vi "DriveModuleControlLogic_ORIG.vi"(8 "Pass_Through_Time":dbl=-1.0 format="%33.4f", 9 "Actual State":T1 {"Angle"."SIN" format="%13.4f"; "Angle"."COS" format="%13.4f"; "Angle"."VALUE" format="%13.4f"}, 10 "Desired State":T1={"Speed"=0.0, "Angle"={"VALUE"=0.0, "COS"=1.0, "SIN"=0.0}} {"Angle"."SIN" format="%13.4f"; "Angle"."COS" format="%13.4f"; "Angle"."VALUE" format="%13.4f"}, 11 "ModualNamePrefix":i32) -> (2 "SpinMotorDmd":dbl, 3 "TravelMotorDmd":dbl)   [LabVIEW 2023]
uses:
  <vilib>/Rock Robotics/WPI/ThirdParty/JAS_Junk/TrajLib/TypeDef/SWERVE_DRIVE_MODULE_STATE.ctl
  <vilib>/Rock Robotics/WPI/ThirdParty/JAS_Junk/TrajLib/TypeDef/ROTATION2D.ctl
  <vilib>/Rock Robotics/WPI/ThirdParty/JAS_Junk/TrajLib/Rotation2d_Minus.vi
  <vilib>/Rock Robotics/WPI/ThirdParty/JAS_Junk/TrajLib/Rotation2d_GetRadians.vi
  <vilib>/Rock Robotics/WPI/ThirdParty/JAS_Junk/TrajLib/SwerveModuleState_New.vi
  <vilib>/Rock Robotics/WPI/ThirdParty/JAS_Junk/TrajLib/Rotation2d_RotateBy.vi
  <vilib>/Rock Robotics/WPI/ThirdParty/JAS_Junk/TrajLib/Rotation2d_CreateAngle.vi
  <vilib>/Rock Robotics/WPI/ThirdParty/JAS_Junk/TrajLib/SimpleMotorFF_Calculate.vi
  <vilib>/Rock Robotics/WPI/ThirdParty/JAS_Junk/TrajLib/PIDController_AtSetpoint.vi
  <vilib>/Rock Robotics/WPI/ThirdParty/JAS_Junk/TrajLib/PIDController_SetPIDF.vi
  <vilib>/Rock Robotics/WPI/ThirdParty/JAS_Junk/TrajLib/PIDController_SetDerivativeFilter.vi
  <vilib>/Rock Robotics/WPI/ThirdParty/JAS_Junk/TrajLib/PIDController_SetIntegratorRange.vi
  <vilib>/Rock Robotics/WPI/ThirdParty/JAS_Junk/TrajLib/PIDController_SetTolerancePandV.vi
  <vilib>/Rock Robotics/WPI/ThirdParty/JAS_Junk/TrajLib/PIDController_DisableContinousInput.vi
  <vilib>/Rock Robotics/WPI/ThirdParty/JAS_Junk/TrajLib/PIDController_EnableContinousInput.vi
  <vilib>/Rock Robotics/WPI/ThirdParty/JAS_Junk/TrajLib/PIDController_Reset.vi
  <vilib>/Rock Robotics/WPI/ThirdParty/JAS_Junk/TrajLib/PIDController_New.vi
  <vilib>/Rock Robotics/WPI/ThirdParty/JAS_Junk/TrajLib/PIDController_SetOutputLimits.vi
  <vilib>/Rock Robotics/WPI/ThirdParty/JAS_Junk/TrajLib/VI/PIDController_SetIntegratorZone.vi
  <vilib>/Rock Robotics/WPI/ThirdParty/JAS_Junk/TrajLib/SlewRateLimiter_New.vi
  <vilib>/Rock Robotics/WPI/ThirdParty/JAS_Junk/TrajLib/SlewRateLimiter_Reset.vi
  <vilib>/Rock Robotics/WPI/ThirdParty/JAS_Junk/TrajLib/SlewRateLimiter_Calculate.vi
  <vilib>/Rock Robotics/WPI/ThirdParty/JAS_Junk/TrajLib/SlewRateLimiter_SetRate.vi
  <vilib>/Rock Robotics/WPI/ThirdParty/JAS_Junk/TrajLib/VI/Util_GetTime_U32.vi
  <vilib>/Rock Robotics/WPI/ThirdParty/JAS_Junk/TrajLib/MathUtil_Clamp.vi
  <vilib>/Rock Robotics/WPI/ThirdParty/JAS_Junk/TrajLib/VI/MathUtil_RateOfChange.vi
  <vilib>/Rock Robotics/WPI/ThirdParty/JAS_Junk/TrajLib/Rotation2d_UnaryMinus.vi
  <vilib>/Rock Robotics/WPI/ThirdParty/JAS_Junk/TrajLib/Rotation2d_CreateXY.vi
  <vilib>/Rock Robotics/WPI/ThirdParty/JAS_Junk/TrajLib/PIDController_NewPeriod.vi
  <vilib>/Rock Robotics/WPI/ThirdParty/JAS_Junk/TrajLib/Util_CalcDist.vi
  <vilib>/Rock Robotics/SystemInterfaces/NetworkCommunication/NetComm_UsageReport_report.vi
  Robot Global Data.vi
  DriveGlobal.vi
  <vilib>/Rock Robotics/WPI/ThirdParty/JAS_Junk/TrajLib/VI/Util_GetTime_U64.vi
  <vilib>/Rock Robotics/WPI/ThirdParty/JAS_Junk/TrajLib/Globals/Util_LibraryGlobals.vi
  <vilib>/Rock Robotics/WPI/ThirdParty/JAS_Junk/TrajLib/PIDController_AdvCalculate_FF_Sp_Pv.vi
  <vilib>/Rock Robotics/WPI/ThirdParty/JAS_Junk/TrajLib/Trajectory_Library.lvlib
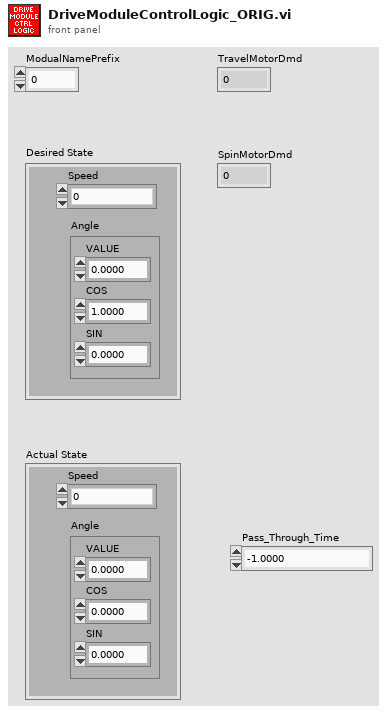
[diagram p1: front panel]
types:
  T1 = typedef "Trajectory_Library.lvlib/SWERVE_DRIVE_MODULE_STATE.ctl" = cluster{"Speed":dbl, "Angle":T2}
  T2 = typedef "Trajectory_Library.lvlib/ROTATION2D.ctl" = cluster{"VALUE":dbl, "COS":dbl, "SIN":dbl}
  T3 = typedef "Trajectory_Library.lvlib/SIMPLE_MOTOR_FF.ctl" = cluster{"Ks":dbl, "Kv":dbl, "Ka":dbl, "KnInv":dbl}
  T4 = typedef "Trajectory_Library.lvlib/PID_ADV_LIMITS.ctl" = cluster{"MaxInput":dbl, "MinInput":dbl, "Continuous":bool, "MaxOutput":dbl, "MinOutput":dbl}
  T5 = typedef "Trajectory_Library.lvlib/PID_ADV_TUNING.ctl" = cluster{"Kf":dbl, "Kp":dbl, "Ki":dbl, "Kd":dbl, "MaximumIntegral":dbl, "MinimumIntegral":dbl, "Filter Derivative":bool, "IntegralZone":dbl}
  T6 = typedef "Trajectory_Library.lvlib/PosCtrl_Tuning_Type.ctl" = cluster{"Slope":dbl, "Offset":dbl, "Error Deadband":dbl, "At Reference Count":i32, "Negate Output":bool, "Max Allowd Position":dbl, "Min Allowd Position":dbl, "Kd":dbl, "FilterDerivative":bool}
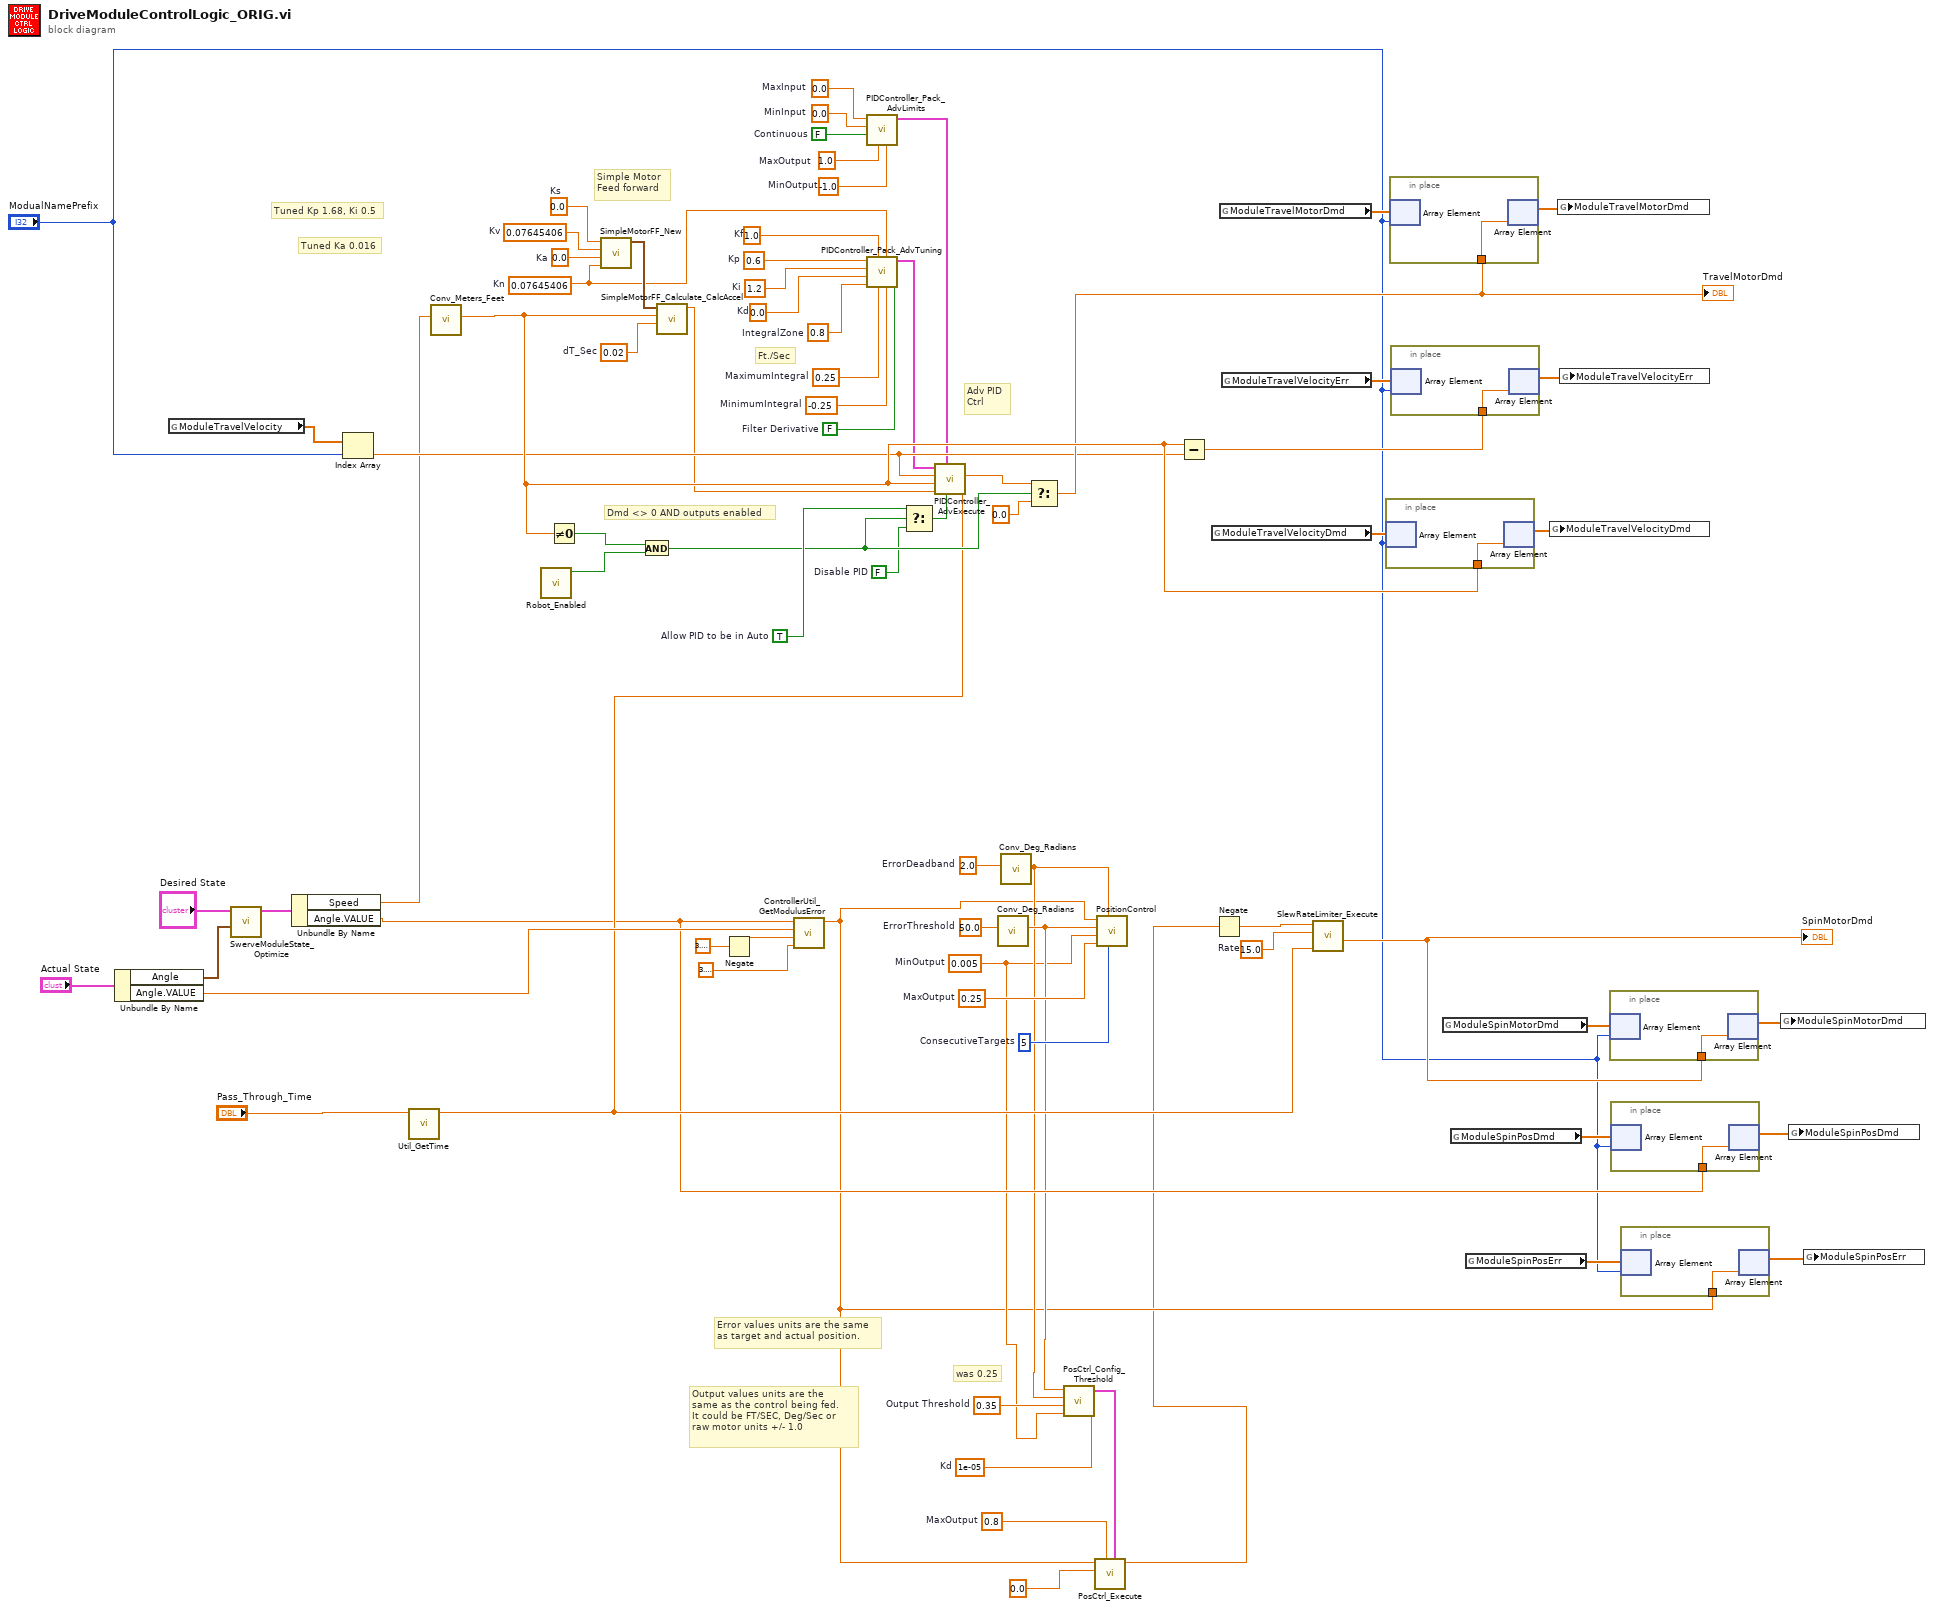
[diagram p0: block diagram]
diagram:
  w10 = 1e-05  # Kd
  w9 = 0.8  # MaxOutput
  w7 = 0.35  # Output Threshold
  w12 = 0.8  # IntegralZone
  w64 = 15.0  # Rate
  w63 = TRUE  # Allow PID to be in Auto
  w61 = FALSE  # Disable PID
  w40 = 0.6  # Kp
  w41 = 1.2  # Ki
  w42 = 0.0  # Kd
  w43 = 1.0  # Kf
  w44 = 0.25  # MaximumIntegral
  w45 = -0.25  # MinimumIntegral
  w46 = FALSE  # Filter Derivative
  w48 = 0.0  # MinInput
  w49 = FALSE  # Continuous
  w50 = 1.0  # MaxOutput
  w47 = -1.0  # MinOutput
  w51 = 0.0  # MaxInput
  w11 = 0.07645406  # Kn
  w35 = 0.02  # dT_Sec
  w37 = 0.0  # Ks
  w38 = 0.07645406  # Kv
  w39 = 0.0  # Ka
  w30 = 5  # ConsecutiveTargets
  w31 = 0.25  # MaxOutput
  w4 = 0.005  # MinOutput
  w33 = 50.0  # ErrorThreshold
  w32 = 2.0  # ErrorDeadband
  # "was 0.25"
  # "Output values units are the\nsame as the control being fed.  \nIt could be FT/SEC, Deg/Sec or\nraw motor units +/- 1.0"
  # "Error values units are the same \nas target and actual position."
  # "Ft./Sec"
  # "Tuned Kp 1.68, Ki 0.5"
  # "Tuned Ka 0.016"
  # "Dmd <> 0 AND outputs enabled"
  # "Adv PID\nCtrl"
  # "Simple Motor\nFeed forward"
  n1 = Unbundle By Name("Actual State") -> ("Angle"=w24:T2, "Angle.VALUE"=w27:dbl)
  n2 = global read "DriveGlobal.vi" "ModuleTravelVelocity"() -> (w55:dbl[])
  n3 = call <vilib>:"SwerveModuleState_Optimize.vi"("CurrentAngle"=w24, "Desired State"="Desired State") -> ("out SWERVE_DRIVE_MODULE_STATE"=w26:T1)  [unwired: 9 in]
  n4 = Unbundle By Name(w26) -> ("Speed"=w34:dbl, "Angle.VALUE"=w16:dbl)
  n5 = Index Array(array=w55, index="ModualNamePrefix") -> (element=w56:dbl)
  n6 = call <vilib>:"Util_GetTime.vi"("Pass_Through_Time"="Pass_Through_Time") -> ("FPGA_Time_Seconds"=w21:dbl)  [unwired: 8 in, 2 out]
  n7 = call <vilib>:"Conv_Meters_Feet.vi"("Meters"=w34) -> ("Feet"=w74:dbl)  [unwired: 10 in]
  n8 = call "Robot_Enabled.vi"() -> ("Robot Enabled"=w19:bool)  [unwired: 11 in]
  n9 = Not Equal To 0?(x=w74) -> (x != 0?=w59:bool)
  n10 = call <vilib>:"SimpleMotorFF_New.vi"("Kn"=w11, "Ka"=w39, "Kv"=w38, "Ks"=w37) -> ("SIMPLE_MOTOR_FF"=w36:T3)  [unwired: 7 in]
  n11 = And(x=w59, y=w19) -> (x .and. y?=w62:bool)
  n12 = call <vilib>:"SimpleMotorFF_Calculate_CalcAccel.vi"("dT_Sec"=w35, "VelSp"=w74, "SIMPLE_MOTOR_FF"=w36) -> ("FeedForward"=w54:dbl)  [unwired: 8 in]
  n13 = Negate(x=3.141592653589793) -> (-x=w25:dbl)
  n14 = call <vilib>:"ControllerUtil_GetModulusError.vi"("Maximum_Input"=3.141592653589793, "Minimum_Input"=w25, "Measurerment(PV)"=w27, "Reference(SP)"=w16) -> ("Error"=w3:dbl)  [unwired: 7 in]
  n15 = call <vilib>:"PIDController_Pack_AdvLimits.vi"("MinOutput"=w47, "MaxOutput"=w50, "Continuous"=w49, "MinInput"=w48, "MaxInput"=w51) -> ("Adv PID Limits"=w53:T4)  [unwired: 6 in]
  n16 = call <vilib>:"PIDController_Pack_AdvTuning.vi"("Filter Derivative"=w46, "MinimumIntegral"=w45, "Kn"=w11, "MaximumIntegral"=w44, "Kf"=w43, "IntegralZone"=w12, "Kd"=w42, "Ki"=w41, "Kp"=w40) -> ("Adv PID Tuning"=w52:T5)  [unwired: 2 in]
  n17 = Select(t=w63, s=w62, f=w61) -> (s? t:f=w60:bool)
  n18 = call <vilib>:"PIDController_AdvExecute.vi"("Time"=w21, "Auto"=w60, "Adv PID Limits"=w53, "FF-FeedForward"=w54, "SP-SetPoint"=w74, "PV-Measurement"=w56, "Adv PID Tuning"=w52) -> ("CO-ControlOutput"=w57:dbl)  [unwired: 2 in, 2 out]
  n19 = call <vilib>:"Conv_Deg_Radians.vi"("Degress"=w33) -> ("Radians"=w6:dbl)  [unwired: 10 in]
  n20 = call <vilib>:"Conv_Deg_Radians.vi"("Degress"=w32) -> ("Radians"=w5:dbl)  [unwired: 10 in]
  n21 = Select(t=w57, s=w62, f=0.0 ("t")) -> (s? t:f=w68:dbl)
  "TravelMotorDmd" <- w68
  n22 = call <vilib>:"PosCtrl_Config_Threshold.vi"("Kd"=w10, "Output Deadband"=w4, "Output Threshold"=w7, "ErrorDeadband"=w5, "ErrorThreshold"=w6) -> ("PosCtrl_Config_Params"=w8:T6)  [unwired: 5 in, 1 out]
  n23 = call <vilib>:"PosCtrl_Execute.vi"("PosCtrl_Config_Params"=w8, "MaxOutput"=w9, "CurrentPosition"=0.0, "TargetPosition"=w3) -> ("Output"=w1:dbl)  [unwired: 5 in, 2 out]
  n24 = call "PositionControl.vi"("ConsecutiveTargets"=w30, "ErrorDeadband"=w5, "MaxOutput"=w31, "MinOutput"=w4, "ErrorThreshold"=w6, "Error"=w3) -> ()  [unwired: 3 in, 3 out]
  n25 = Subtract(x=w74, y=w56) -> (x-y=w71:dbl)
  n26 = global read "DriveGlobal.vi" "ModuleTravelVelocityDmd"() -> (w72:dbl[])
  n27 = Negate(x=w1) -> (-x=w65:dbl)
  n28 = global read "DriveGlobal.vi" "ModuleTravelMotorDmd"() -> (w66:dbl[])
  n29 = global read "DriveGlobal.vi" "ModuleTravelVelocityErr"() -> (w69:dbl[])
  n30 = call <vilib>:"SlewRateLimiter_Execute.vi"("Time"=w21, "PositiveRate"=w64, "Input"=w65) -> ("Output"=w77:dbl)  [unwired: 7 in, 1 out]
  "SpinMotorDmd" <- w77
  n31 = in-place {
    in-place-border: w74 -> [w78]
    n32 = in-place-array #1(w72, "ModualNamePrefix") -> ()  [unwired: 1 out]
    n33 = in-place-array #1(w78) -> (w73:dbl[])  [unwired: 1 out]
  }
  n34 = in-place {
    in-place-border: w68 -> [w79]
    n35 = in-place-array #2(w66, "ModualNamePrefix") -> ()  [unwired: 1 out]
    n36 = in-place-array #2(w79) -> (w67:dbl[])  [unwired: 1 out]
  }
  n37 = in-place {
    in-place-border: w71 -> [w80]
    n38 = in-place-array #3(w69, "ModualNamePrefix") -> ()  [unwired: 1 out]
    n39 = in-place-array #3(w80) -> (w70:dbl[])  [unwired: 1 out]
  }
  n40 = global read "DriveGlobal.vi" "ModuleSpinMotorDmd"() -> (w75:dbl[])
  n41 = global read "DriveGlobal.vi" "ModuleSpinPosDmd"() -> (w17:dbl[])
  n42 = global read "DriveGlobal.vi" "ModuleSpinPosErr"() -> (w14:dbl[])
  n43 = global write "DriveGlobal.vi" "ModuleTravelVelocityDmd"(w73) -> ()
  n44 = global write "DriveGlobal.vi" "ModuleTravelMotorDmd"(w67) -> ()
  n45 = global write "DriveGlobal.vi" "ModuleTravelVelocityErr"(w70) -> ()
  n46 = in-place {
    in-place-border: w77 -> [w81]
    n47 = in-place-array #4(w75, "ModualNamePrefix") -> ()  [unwired: 1 out]
    n48 = in-place-array #4(w81) -> (w76:dbl[])  [unwired: 1 out]
  }
  n49 = in-place {
    in-place-border: w16 -> [w82]
    n50 = in-place-array #5(w17, "ModualNamePrefix") -> ()  [unwired: 1 out]
    n51 = in-place-array #5(w82) -> (w18:dbl[])  [unwired: 1 out]
  }
  n52 = in-place {
    in-place-border: w3 -> [w83]
    n53 = in-place-array #6(w14, "ModualNamePrefix") -> ()  [unwired: 1 out]
    n54 = in-place-array #6(w83) -> (w15:dbl[])  [unwired: 1 out]
  }
  n55 = global write "DriveGlobal.vi" "ModuleSpinMotorDmd"(w76) -> ()
  n56 = global write "DriveGlobal.vi" "ModuleSpinPosDmd"(w18) -> ()
  n57 = global write "DriveGlobal.vi" "ModuleSpinPosErr"(w15) -> ()
